vi "校准设置页.vi"() -> ()   [LabVIEW 2016, in "斯坦道CODMn.lvlib"]
uses:
  <vilib>/Analysis/6fits.llb/Curve Fitting Criteria.ctl
  <vilib>/Analysis/NI_AALPro.lvlib
  <vilib>/ptbypt/NI_PtbyPt.lvlib
panel:
  in  "读取公式":bool
  in  "历史数据导入":T1(radio)
  out "校准任务":bool
  in  "二次方程2":cluster{"K":dbl, "B":dbl, "x^2":dbl} {"x^2" format="%#.6g"; "K" format="%#.6g"; "B" format="%#.6g"}
  in  "公式切换阈值滴定数(0~9999)":dbl
  out "校准状态":T2(ring)
  out "模型刷新":bool
  in  "校准按钮":T1(radio)
  in  "校准导入":bool
  in  "曲线模型":T3={"标液浓度1"=0.0, "测量吸光度1"=0.0, "样品1启用"=FALSE, "标液浓度2"=0.0, "测量吸光度2"=0.0, "样品2启用"=FALSE, "标液浓度3"=0.0, "测量吸光度3"=0.0, "样品3启用"=FALSE, "标液浓度4"=0.0, "测量吸光度4"=0.0, "样品4启用"=FALSE, "标液浓度5"=0.0, "测量吸光度5"=0.0, "样品5启用"=FALSE, "模型"=enum."线性", "精度"=4.0, "XY图"=[], "拟合公式"="", "r^2"=0.0, "标样一校准时间"=timestamp(0 s since 1904-01-01), "标样二校准时间"=timestamp(0 s since 1904-01-01), "标样三校准时间"=timestamp(0 s since 1904-01-01), "标样四校准时间"=timestamp(0 s since 1904-01-01), "标样五校准时间"=timestamp(0 s since 1904-01-01), "二次方程"={"K"=0.0, "B"=0.0, "x^2"=0.0}, "标定时间"=timestamp(0 s since 1904-01-01), "拟合公式 2"="", "r^2 2"=0.0} {"r^2 2" format="%.7f"; "标定时间" format="%<%Y/%m/%d %H:%M:%S>T"; "二次方程"."x^2" format="%#.6g"; "二次方程"."K" format="%#.6g"; "二次方程"."B" format="%#.6g"; "标样五校准时间" format="%<%Y/%m/%d %H:%M:%S>T"; "标样四校准时间" format="%<%Y/%m/%d %H:%M:%S>T"; "标样三校准时间" format="%<%Y/%m/%d %H:%M:%S>T"; "标样二校准时间" format="%<%Y/%m/%d %H:%M:%S>T"; "标样一校准时间" format="%<%Y/%m/%d %H:%M:%S>T"; "r^2" format="%.7f"; "测量吸光度5" format="%#.6f"; "测量吸光度4" format="%#.6f"; "测量吸光度3" format="%#.6f"; "测量吸光度2" format="%#.6f"; "测量吸光度1" format="%#.6f"}
  in  "测量模式":T4(ring)
  in  "参数下拉列表":u16(ring) items=["CODMn"=21]
  in  "量程下拉列表":enum16{"低量程", "高量程"}(ring)
  # "校准时间"
  # "标液浓度"
  # "滴定数"
  # "标液一"
  # "标液二"
  # "标液三"
  # "零点"
  # "跨度"
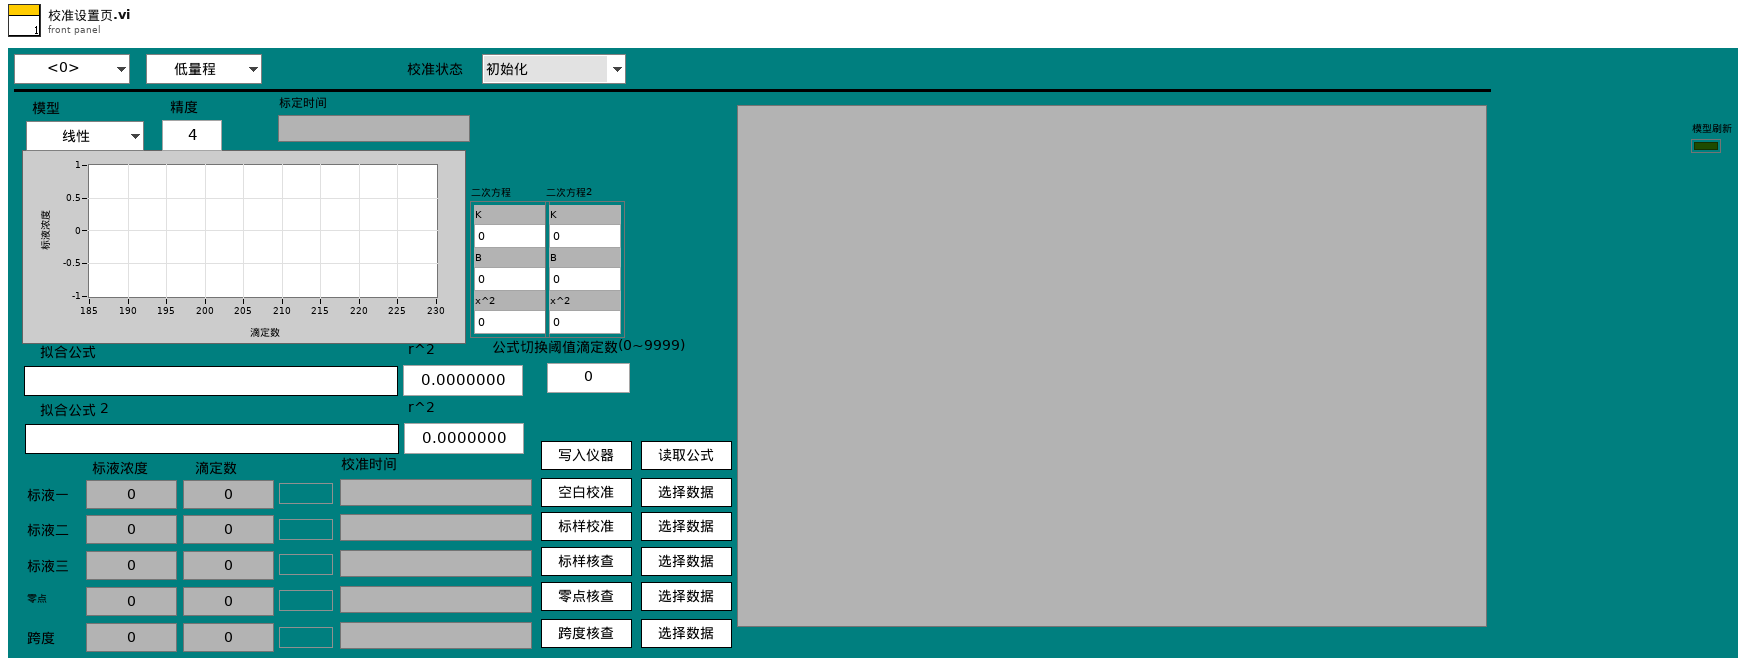
[diagram p1: front panel]
types:
  T1 = enum32{"未选择", "空白校准", "标样校准", "标样核查", "零点核查", "跨度核查"}
  T2 = enum16{"初始化", "解析数据", "判断任务类型", "执行测试任务", "等待测试任务完成", "获取测试数据", "任务结束判定", "计算公式", "结束"}
  T3 = cluster{"标液浓度1":dbl, "测量吸光度1":dbl, "样品1启用":bool, "标液浓度2":dbl, "测量吸光度2":dbl, "样品2启用":bool, "标液浓度3":dbl, "测量吸光度3":dbl, "样品3启用":bool, "标液浓度4":dbl, "测量吸光度4":dbl, "样品4启用":bool, "标液浓度5":dbl, "测量吸光度5":dbl, "样品5启用":bool, "模型":enum32{"线性", "多项式", "折线"}, "精度":dbl, "XY图":cluster{"X Values":dbl[], "Y Values":dbl[]}[], "拟合公式":string, "r^2":dbl, "标样一校准时间":timestamp, "标样二校准时间":timestamp, "标样三校准时间":timestamp, "标样四校准时间":timestamp, "标样五校准时间":timestamp, "二次方程":cluster{"K":dbl, "B":dbl, "x^2":dbl}, "标定时间":timestamp, "拟合公式 2":string, "r^2 2":dbl}
  T4 = enum16{"", "水样测量", "标样核查", "零点核查", "跨度核查", "空白测试", "平行样测试", "加标回收", "空白校准", "标样校准"}
  T5 = typedef "斯坦道CODMn.lvlib/校准任务.ctl" = cluster{"id":u16, "任务类型":enum16{"未选择", "空白校准", "标样校准", "标样核查", "零点核查", "跨度核查"}, "量程下拉列表":enum16{"低量程", "高量程"}, "状态":enum16{"已执行", "待执行", "执行中", "停止"}, "标液浓度":dbl, "吸光值":dbl, "校准时间":timestamp, "报警状态":enum16{"正常数据", "报警数据"}}
  T6 = cluster{"数组 2[0]":sgl, "数组 2[1]":sgl, "数组 2[2]":sgl, "数组 2[3]":sgl, "数组 2[4]":sgl, "数组 2[5]":sgl, "数组 2[6]":sgl, "数组 2[7]":sgl, "数组 2[8]":sgl, "数组 2[9]":sgl, "数组 2[10]":sgl, "数组 2[11]":sgl, "数组 2[12]":sgl, "数组 2[13]":sgl, "数组 2[14]":sgl, "数组 2[15]":sgl, "数组 2[16]":sgl, "数组 2[17]":sgl, "数组 2[18]":sgl, "数组 2[19]":sgl, "数组 2[20]":sgl, "数组 2[21]":sgl, "数组 2[22]":sgl, "数组 2[23]":sgl, "数组 2[24]":sgl, "数组 2[25]":sgl, "数组 2[26]":sgl, "数组 2[27]":sgl, "数组 2[28]":sgl, "数组 2[29]":sgl, "数组 2[30]":sgl, "数组 2[31]":sgl, "数组 2[32]":sgl, "数组 2[33]":sgl, "数组 2[34]":sgl, "数组 2[35]":sgl, "数组 2[36]":sgl, "数组 2[37]":sgl, "数组 2[38]":sgl, "数组 2[39]":sgl, "数组 2[40]":sgl, "数组 2[41]":sgl}
  T7 = cluster{"标液浓度1":dbl, "测量吸光度1":dbl, "样品1启用":bool, "标液浓度2":dbl, "测量吸光度2":dbl, "样品2启用":bool, "标液浓度3":dbl, "测量吸光度3":dbl, "样品3启用":bool, "标液浓度4":dbl, "测量吸光度4":dbl, "样品4启用":bool, "标液浓度5":dbl, "测量吸光度5":dbl, "样品5启用":bool, "模型":enum32{"线性", "多项式", "折线"}, "精度":dbl, "XY图":cluster{"X Values":dbl[], "Y Values":dbl[]}[], "拟合公式":string, "r^2":dbl, "标样一校准时间":timestamp, "标样二校准时间":timestamp, "标样三校准时间":timestamp, "标样四校准时间":timestamp, "标样五校准时间":timestamp, "二次方程":cluster{"c":dbl, "x":dbl, "x^2":dbl}, "标定时间":timestamp, "拟合公式 2":string, "r^2 2":dbl}[][]
  T8 = cluster{"标液浓度1":dbl, "测量吸光度1":dbl, "样品1启用":bool, "标液浓度2":dbl, "测量吸光度2":dbl, "样品2启用":bool, "标液浓度3":dbl, "测量吸光度3":dbl, "样品3启用":bool, "标液浓度4":dbl, "测量吸光度4":dbl, "样品4启用":bool, "标液浓度5":dbl, "测量吸光度5":dbl, "样品5启用":bool, "模型":enum32{"线性", "多项式", "折线"}, "精度":dbl, "XY图":cluster{"X Values":dbl[], "Y Values":dbl[]}[], "拟合公式":string, "r^2":dbl, "标样一校准时间":timestamp, "标样二校准时间":timestamp, "标样三校准时间":timestamp, "标样四校准时间":timestamp, "标样五校准时间":timestamp, "二次方程":cluster{"c":dbl, "x":dbl, "x^2":dbl}, "标定时间":timestamp, "拟合公式 2":string, "r^2 2":dbl}
  T9 = typedef "NI_AALPro.lvlib/Curve Fitting Criteria.ctl" = u16
  T10 = enum32{"Bad", "Idle", "Run top level", "Running"}
  T11 = cluster{"时间":timestamp, "标液值":dbl, "检测值":dbl, "吸光值":dbl}
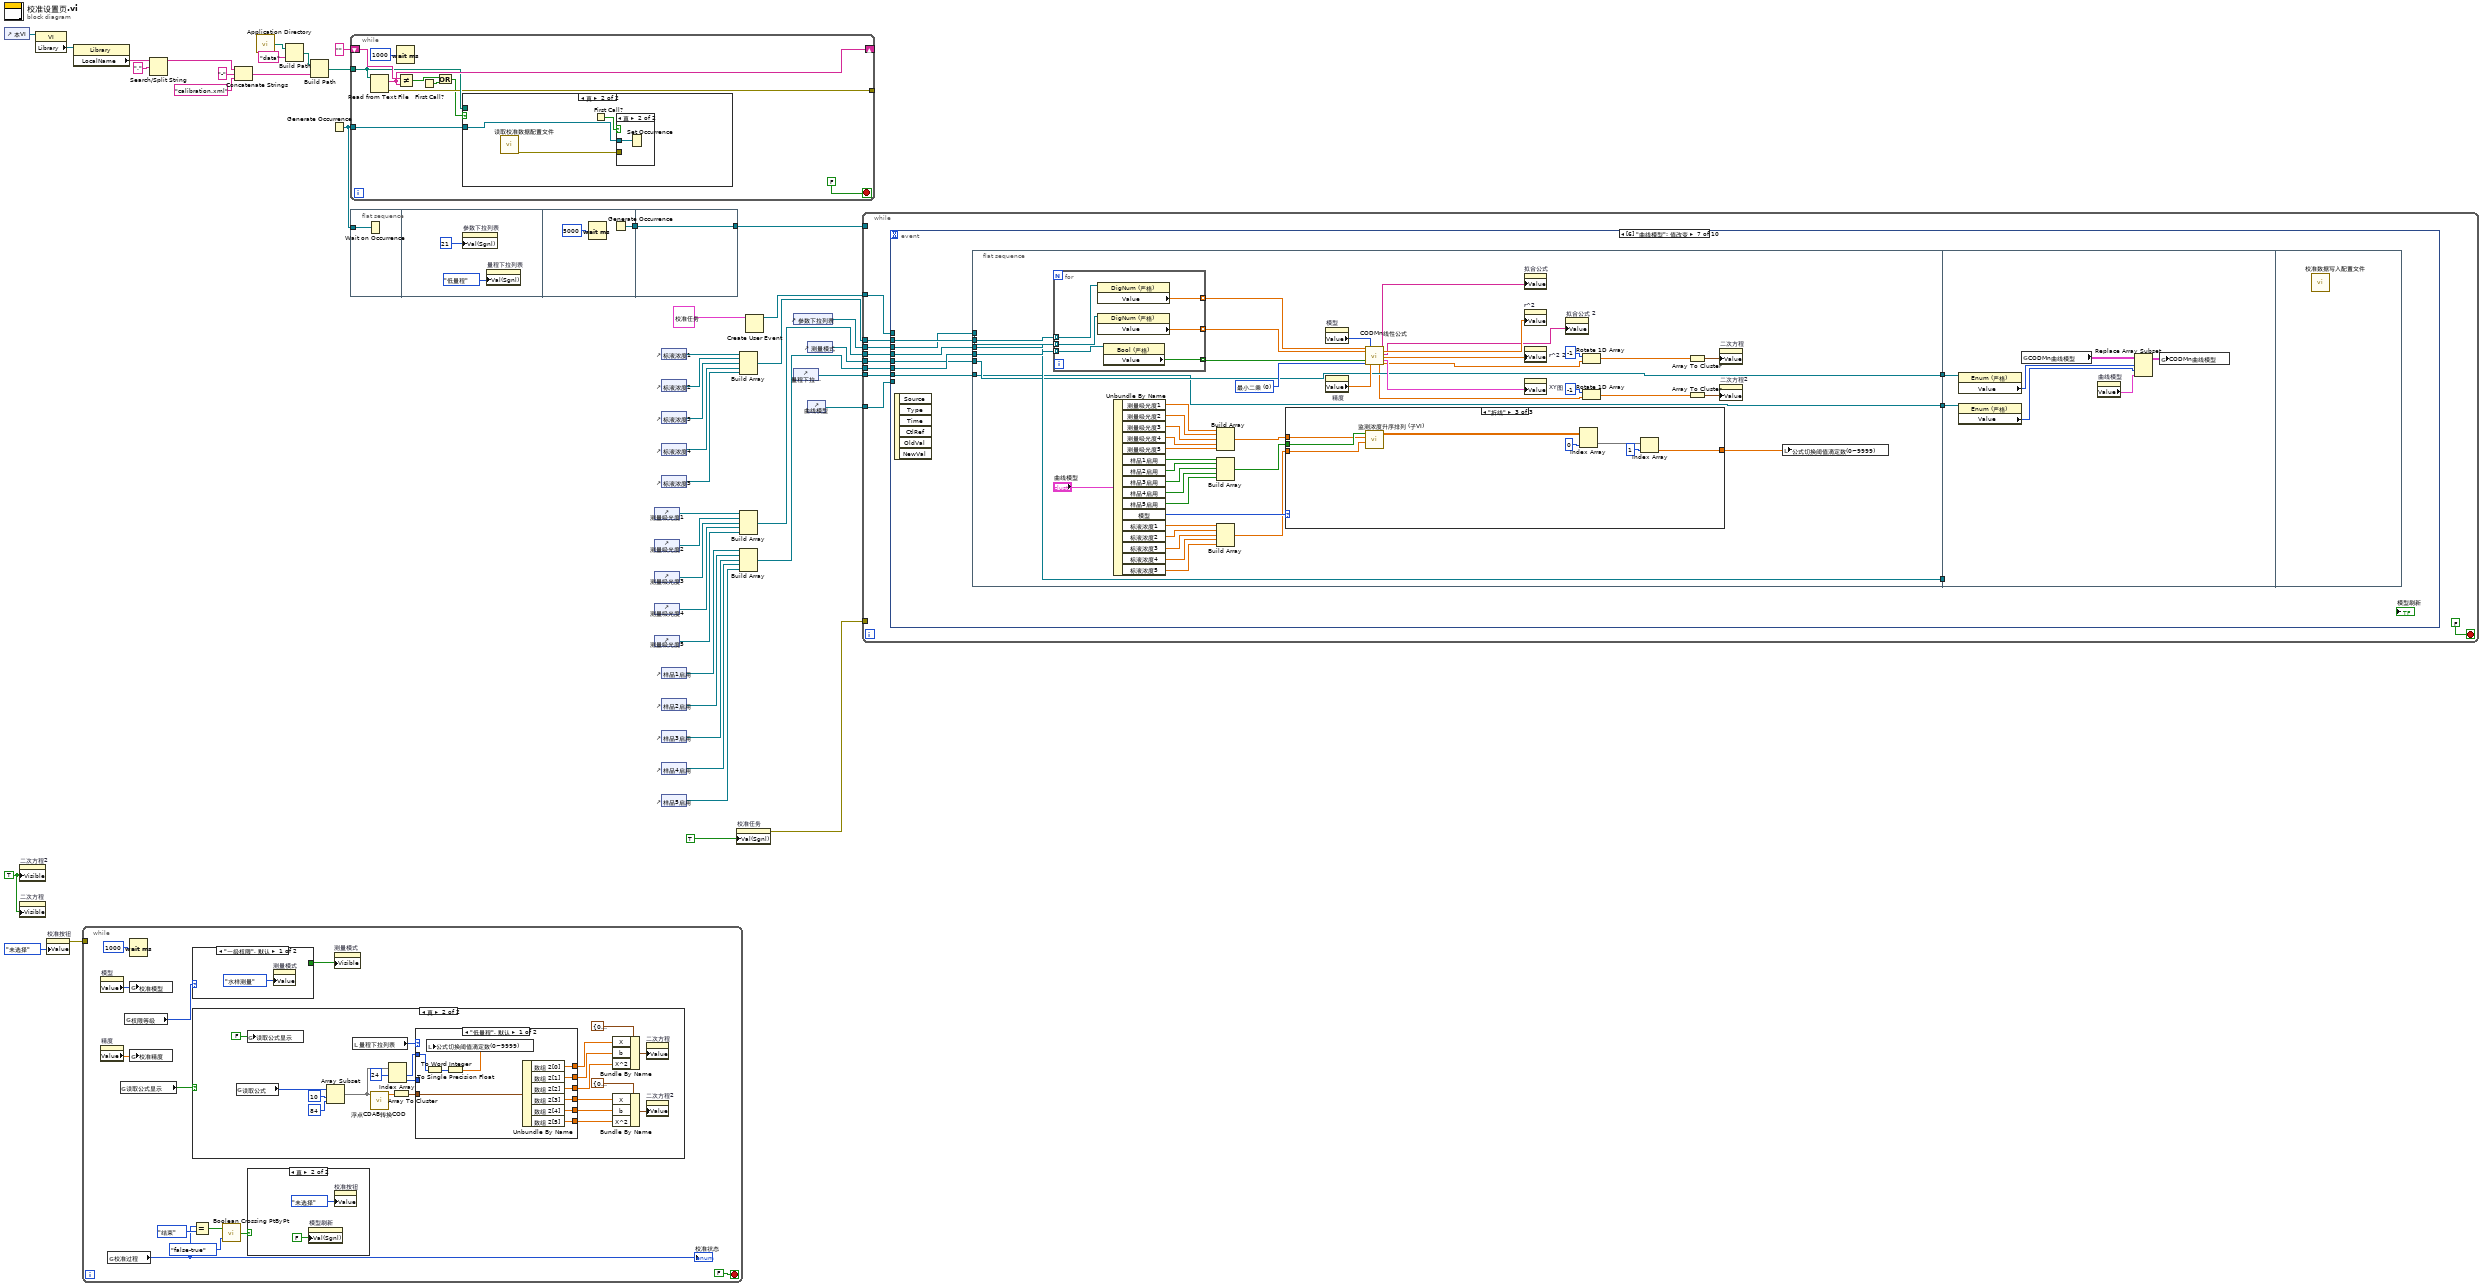
[diagram p0: block diagram]
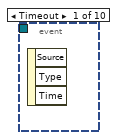
[diagram p4: hidden frame]
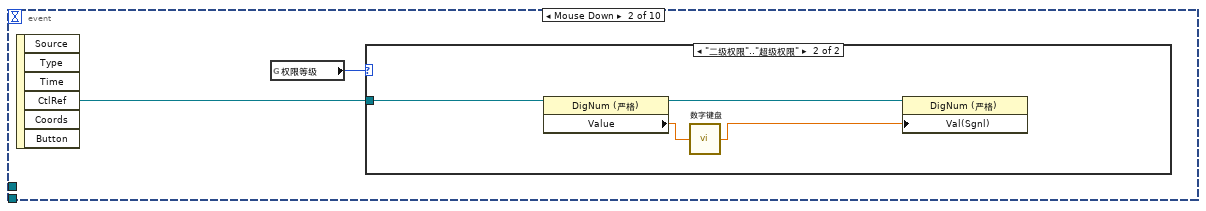
[diagram p5: hidden frame]
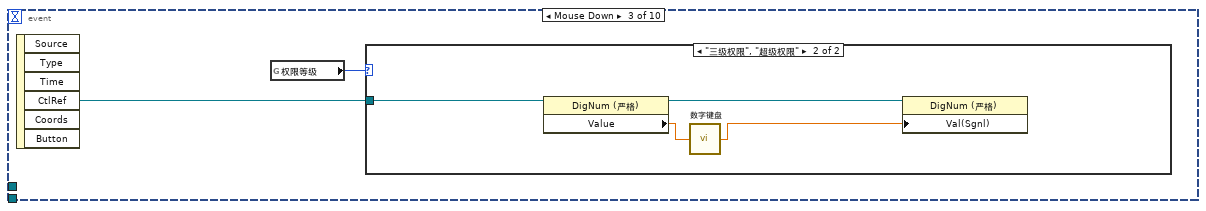
[diagram p7: hidden frame]
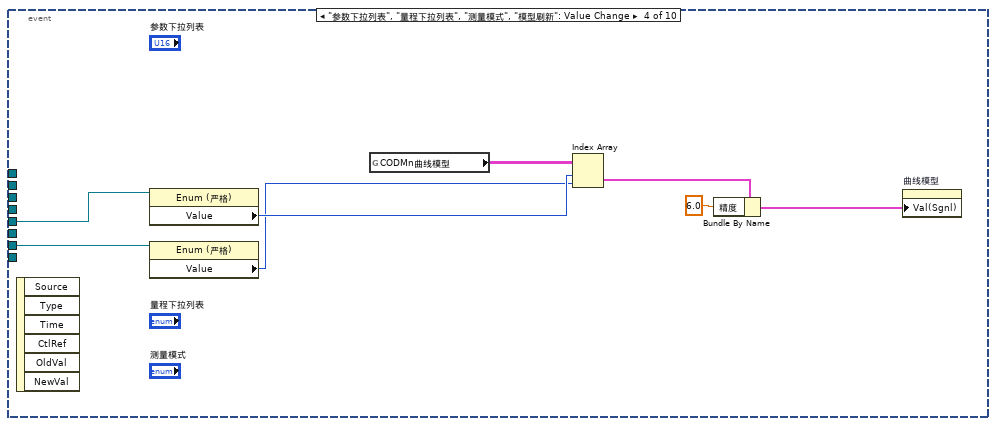
[diagram p9: hidden frame]
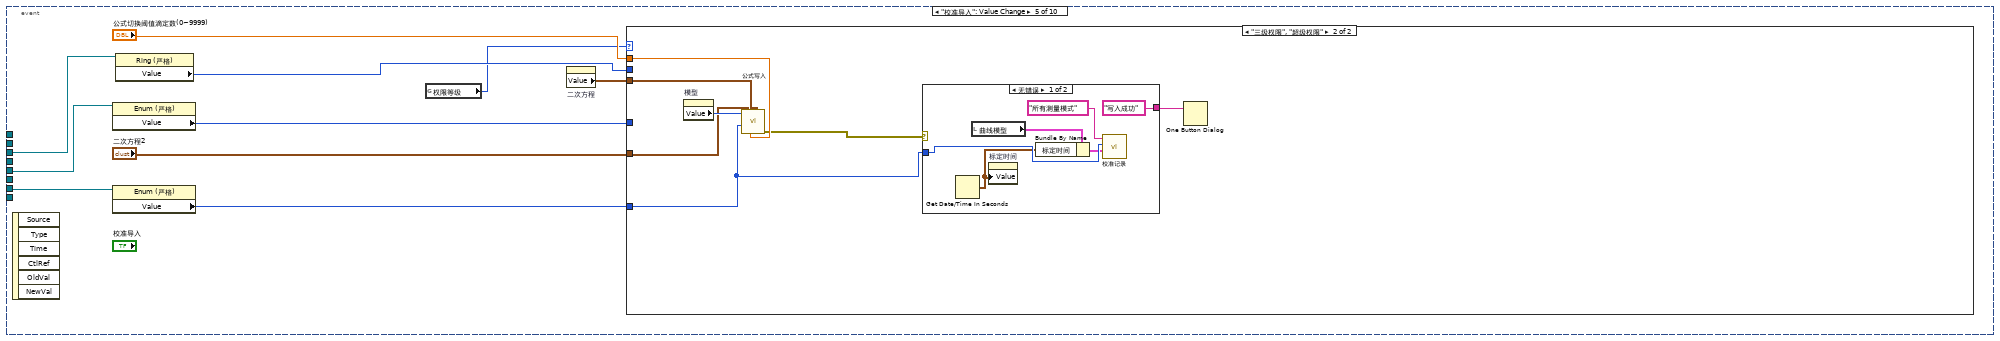
[diagram p10: hidden frame]
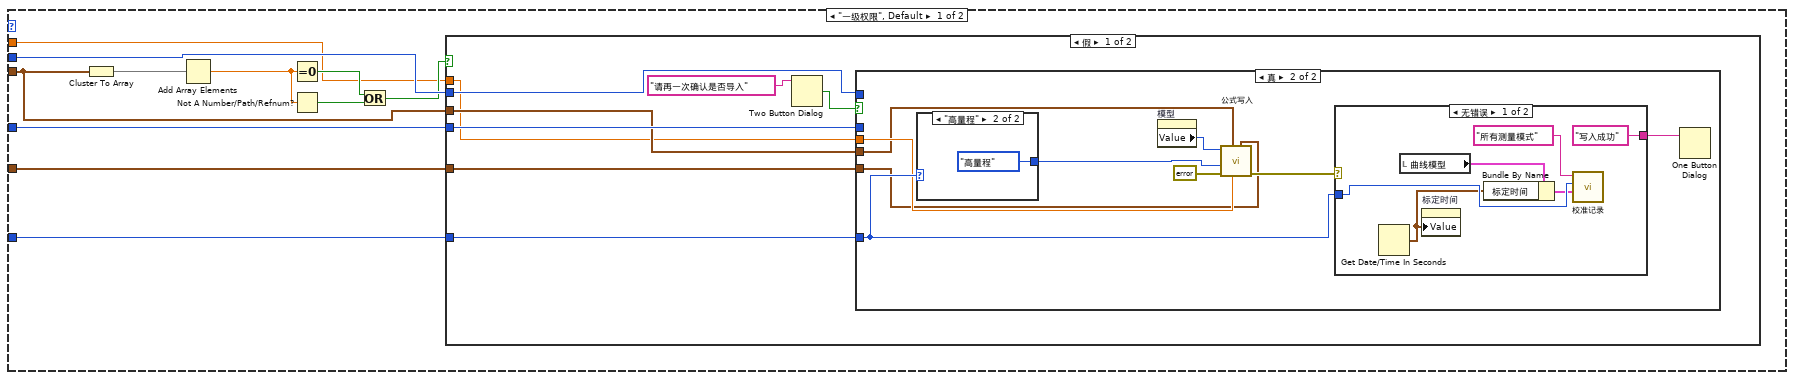
[diagram p11: hidden frame]
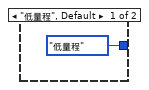
[diagram p13: hidden frame]
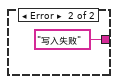
[diagram p14: hidden frame]
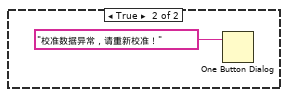
[diagram p15: hidden frame]
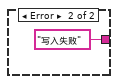
[diagram p16: hidden frame]
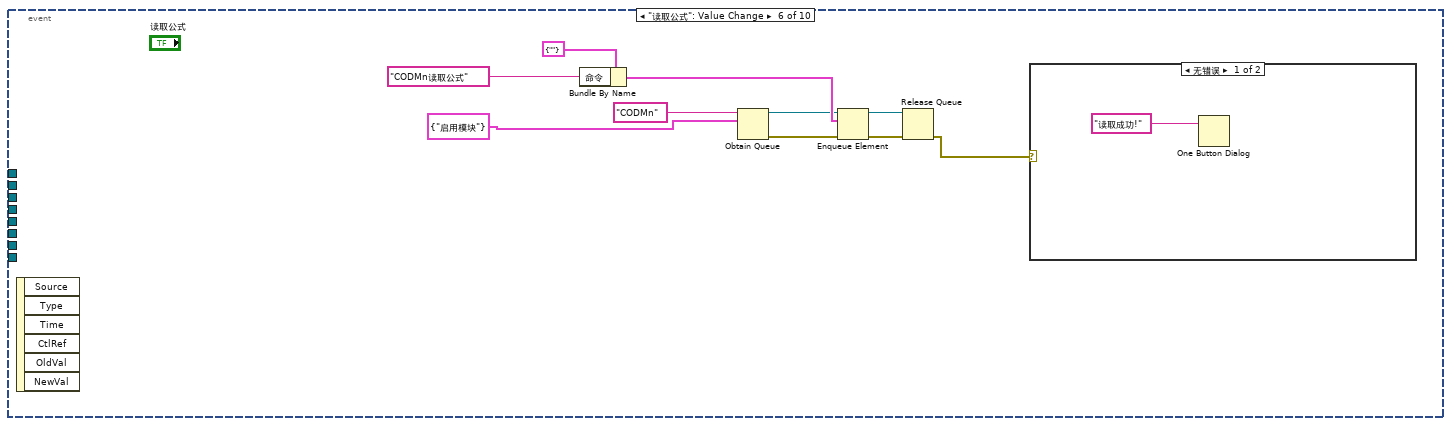
[diagram p17: hidden frame]
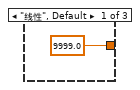
[diagram p19: hidden frame]
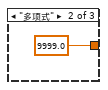
[diagram p20: hidden frame]
diagram:
  w2 = TRUE ("可见")
  n1 = control-ref of="本VI"() -> (w9:refnum<vi>)
  n2 = property on="二次方程2" class="Clust (严格)"("Visible"=w2) -> ()  [unwired: 2 in, 2 out]
  n3 = property on="二次方程" class="Clust (严格)"("Visible"=w2) -> ()  [unwired: 2 in, 2 out]
  n4 = property class="VI"(reference=w9) -> ("Library"=w18:refnum<vi>)  [unwired: 1 in, 2 out]
  n5 = property on="校准按钮" class="RadioBtnsControl (严格)"("Value"=T1."未选择" ("校准按钮")) -> (error out=w1:errorcluster)  [unwired: 2 in, 1 out]
  n6 = property class="Library"(reference=w18) -> ("LocalName"=w16:string)  [unwired: 1 in, 2 out]
  n7 = while {
    tunnel: w1 -> [_]
    stop <- FALSE stop-if-true
    n8 = property on="模型" class="Enum (严格)"() -> ("Value"=w49:enum32{"线性", "多项式", "折线"})  [unwired: 2 in, 2 out]
    n9 = property on="精度" class="DigNum (严格)"() -> ("Value"=w48:dbl)  [unwired: 2 in, 2 out]
    n10 = global read "校准数据全局变量.vi" "校准过程"() -> (w50:T2)
    "校准状态" <- w50
    n11 = global read "COD内部交互全局.vi" "读取公式显示"() -> (w46:bool)
    n12 = global read "CODMN外部API.vi" "权限等级"() -> (w47:enum16{"一级权限", "二级权限", "三级权限", "超级权限"})
    n13 = Wait (ms)(milliseconds to wait=u32 1000 ("等待时间（毫秒）")) -> ()  [unwired: 1 out]
    n14 = global write "校准数据全局变量.vi" "校准模型"(w49) -> ()
    n15 = global write "校准数据全局变量.vi" "校准精度"(w48) -> ()
    n16 = case shown="\"一级权限\", 默认" w47 {
      tunnel: [_ TRUE ("可见")] -> w55
      frame "一级权限", Default {
        n17 = property on="测量模式" class="Enum (严格)"("Value"=T4."水样测量" ("测量模式")) -> ()  [unwired: 2 in, 2 out]
      }
      frame "三级权限", "超级权限" {
      }
    }
    n18 = case shown="真" w46 {
      frame False {
      }
      frame True {
        n19 = global read "COD内部交互全局.vi" "读取公式"() -> (w72:u16[])
        n20 = global write "COD内部交互全局.vi" "读取公式显示"(FALSE ("读取公式显示")) -> ()
        n21 = Array Subset(array=w72, index=10 ("索引"), length=84 ("长度")) -> (w74:u16[])
        n22 = local read "量程下拉列表"() -> (w71:enum16{"低量程", "高量程"})
        n23 = call "浮点CDAB转换COD.vi"("数组"=w74) -> ("数组 2"=w77:sgl[])  [unwired: 10 in]
        n24 = Index Array(array=w74, index #1=24 ("索引")) -> (element #1=w68:u16, element #2=w69:u16)  [unwired: 1 in]
        n25 = Array To Cluster(array=w77) -> (cluster=w70:T6)
        n26 = case shown="\"低量程\", 默认" w71 {
          tunnel: w70 -> [w88 w98]
          tunnel: w69 -> [_ _]
          tunnel: w68 -> [w80 w90]
          tunnel: [w87 w97] -> w65
          tunnel: [w86 w96] -> w64
          tunnel: [w85 w95] -> w63
          tunnel: [w84 w94] -> w62
          tunnel: [w83 w93] -> w61
          tunnel: [w82 w92] -> w60
          frame "低量程", Default {
            n27 = To Word Integer(number=w80) -> (16bit integer=w81:i16)
            n28 = To Single Precision Float(number=w81) -> (single precision float=w79:sgl)
            n29 = local write "公式切换阈值滴定数(0~9999)"(w79) -> ()
            n30 = Unbundle By Name(w88) -> ("数组 2[0]"=w87:sgl, "数组 2[1]"=w86:sgl, "数组 2[2]"=w85:sgl, "数组 2[3]"=w84:sgl, "数组 2[4]"=w83:sgl, "数组 2[5]"=w82:sgl)
          }
          frame "高量程" {
            n31 = To Word Integer(number=w90) -> (16bit integer=w91:i16)
            n32 = To Single Precision Float(number=w91) -> (single precision float=w89:sgl)
            n33 = local write "公式切换阈值滴定数(0~9999)"(w89) -> ()
            n34 = Unbundle By Name(w98) -> ("数组 2[6]"=w97:sgl, "数组 2[7]"=w96:sgl, "数组 2[8]"=w95:sgl, "数组 2[9]"=w94:sgl, "数组 2[10]"=w93:sgl, "数组 2[11]"=w92:sgl)
          }
        }
        n35 = Bundle By Name(cluster=cluster{"X":dbl, "b":dbl, "X^2":dbl} {"X"=0.0, "b"=0.0, "X^2"=0.0} ("方程系数"), "X"=w65, "b"=w64, "X^2"=w63) -> (w59:cluster{"X":dbl, "b":dbl, "X^2":dbl})
        n36 = Bundle By Name(cluster=cluster{"X":dbl, "b":dbl, "X^2":dbl} {"X"=0.0, "b"=0.0, "X^2"=0.0} ("方程系数"), "X"=w62, "b"=w61, "X^2"=w60) -> (w58:cluster{"X":dbl, "b":dbl, "X^2":dbl})
        n37 = property on="二次方程" class="Clust (严格)"("Value"=w59) -> ()  [unwired: 2 in, 2 out]
        n38 = property on="二次方程2" class="Clust (严格)"("Value"=w58) -> ()  [unwired: 2 in, 2 out]
      }
    }
    n39 = Equal?(x=w50, y=T2."结束" ("校准过程")) -> (x = y?=w54:bool)
    n40 = call <vilib>:"Boolean Crossing PtByPt.vi"("direction"=enum16{"either", "false-true", "true-false"}."false-true", "input"=w54) -> ("crossing"=w52:bool)  [unwired: 1 in]
    n41 = case shown="真" w52 {
      frame False {
      }
      frame True {
        n42 = property on="模型刷新" class="Bool (严格)"("Val(Sgnl)"=FALSE ("值(信号)")) -> ()  [unwired: 2 in, 2 out]
        n43 = property on="校准按钮" class="RadioBtnsControl (严格)"("Value"=T1."未选择" ("校准按钮")) -> ()  [unwired: 2 in, 2 out]
      }
    }
    n44 = property on="测量模式" class="Enum (严格)"("Visible"=w55) -> ()  [unwired: 2 in, 2 out]
  }
  n45 = Search/Split String(string=w16, search string/char (-)="." ("搜索字符串/字符(-)")) -> (substring before match=w14:string)  [unwired: 1 in, 2 out]
  n46 = Concatenate Strings(w14, "-" ("字符串"), "calibration.xml" ("名称或相对路径")) -> (w11:string)
  n47 = call <vilib>:"Application Directory.vi"() -> ("Application Directory"=w19:path)
  n48 = Build Path(base path=w19, name or relative path="data" ("名称或相对路径")) -> (appended path=w17:path)
  n49 = Build Path(base path=w17, name or relative path=w11) -> (appended path=w10:path)
  n50 = Generate Occurrence() -> (w7:refnum<k4>)
  n51 = while {
    shift-right: [w110] -> _
    shift-left: "" -> [w111]
    tunnel: w10 -> [w109]
    tunnel: [w107] -> _
    tunnel: w7 -> [w103]
    stop <- FALSE stop-if-true
    n52 = Read from Text File(file (use dialog)=w109) -> (text=w110:string, error out=w107:errorcluster)  [unwired: 3 in, 2 out]
    n53 = Wait (ms)(milliseconds to wait=u32 1000 ("等待时间（毫秒）")) -> ()  [unwired: 1 out]
    n54 = Not Equal?(x=w111, y=w110) -> (x != y?=w105:bool)
    n55 = First Call?() -> (First Call?: T/F=w106:bool)
    n56 = Or(x=w105, y=w106) -> (x .or. y?=w104:bool)
    n57 = case shown="真" w104 {
      tunnel: w109 -> [_ _]
      tunnel: w103 -> [_ w114]
      frame False {
      }
      frame True {
        n58 = call "读取校准数据配置文件.vi"() -> ("错误输出"=w113:errorcluster)  [unwired: 11 in]
        n59 = First Call?() -> (First Call?: T/F=w115:bool)
        n60 = case shown="真" w115 {
          tunnel: w114 -> [_ w116]
          tunnel: w113 -> [_ _]
          frame False {
          }
          frame True {
            n61 = Set Occurrence(w116) -> ()
          }
        }
      }
    }
  }
  n62 = flat-sequence {
    tunnel: w7 -> [w117]
    tunnel: [w121] -> w45
    tunnel: [w122] -> w44
    tunnel: w45 -> [w122]
    frame #0 {
      n63 = Wait on Occurrence(2:w117) -> ()  [unwired: 2 in, 1 out]
    }
    frame #1 {
      n64 = property on="参数下拉列表" class="Ring (严格)"("Val(Sgnl)"=u16 21 ("值(信号)")) -> ()  [unwired: 2 in, 2 out]
      n65 = property on="量程下拉列表" class="Enum (严格)"("Val(Sgnl)"=enum16{"低量程", "高量程"}."低量程" ("值(信号)")) -> ()  [unwired: 2 in, 2 out]
    }
    frame #2 {
      n66 = Wait (ms)(milliseconds to wait=u32 5000 ("等待时间（毫秒）")) -> ()  [unwired: 1 out]
      n67 = Generate Occurrence() -> (w121:refnum<k4>)
    }
    frame #3 {
    }
  }
  n68 = control-ref of="测量吸光度1"() -> (w32:refnum<vi>)
  n69 = control-ref of="测量吸光度2"() -> (w33:refnum<vi>)
  n70 = control-ref of="测量吸光度3"() -> (w34:refnum<vi>)
  n71 = control-ref of="测量吸光度4"() -> (w35:refnum<vi>)
  n72 = control-ref of="测量吸光度5"() -> (w36:refnum<vi>)
  n73 = control-ref of="标液浓度1"() -> (w30:refnum<vi>)
  n74 = control-ref of="标液浓度2"() -> (w29:refnum<vi>)
  n75 = control-ref of="标液浓度3"() -> (w28:refnum<vi>)
  n76 = control-ref of="标液浓度4"() -> (w27:refnum<vi>)
  n77 = control-ref of="标液浓度5"() -> (w26:refnum<vi>)
  n78 = control-ref of="样品1启用"() -> (w42:refnum<vi>)
  n79 = control-ref of="样品2启用"() -> (w41:refnum<vi>)
  n80 = control-ref of="样品3启用"() -> (w40:refnum<vi>)
  n81 = control-ref of="样品4启用"() -> (w39:refnum<vi>)
  n82 = control-ref of="样品5启用"() -> (w38:refnum<vi>)
  n83 = property on="校准任务" class="Bool (严格)"("Val(Sgnl)"=TRUE ("值(信号)")) -> (error out=w5:errorcluster)  [unwired: 2 in, 1 out]
  n84 = Build Array(w30, w29, w28, w27, w26) -> (w25:refnum<vi>[])
  n85 = Build Array(w32, w33, w34, w35, w36) -> (w31:refnum<vi>[])
  n86 = Build Array(w42, w41, w40, w39, w38) -> (w37:refnum<vi>[])
  n87 = Create User Event(user event datatype=T5 {"id"=0, "任务类型"=enum."未选择", "量程下拉列表"=enum."低量程", "状态"=enum."已执行", "标液浓度"=0.0, "吸光值"=0.0, "校准时间"=timestamp(0 s since 1904-01-01), "报警状态"=enum."正常数据"} ("校准任务")) -> (user event=w3:refnum<user-event>)  [unwired: 1 in, 1 out]
  n88 = control-ref of="参数下拉列表"() -> (w43:refnum<vi>)
  n89 = control-ref of="量程下拉列表"() -> (w23:refnum<vi>)
  n90 = control-ref of="测量模式"() -> (w24:refnum<vi>)
  n91 = control-ref of="曲线模型"() -> (w21:refnum<vi>)
  n92 = while {
    tunnel: w44 -> [_]
    tunnel: w43 -> [w130]
    tunnel: w37 -> [w129]
    tunnel: w31 -> [w128]
    tunnel: w25 -> [w127]
    tunnel: w24 -> [w126]
    tunnel: w23 -> [w125]
    tunnel: w21 -> [w124]
    tunnel: w5 -> [_]
    tunnel: w3 -> [w123]
    stop <- FALSE stop-if-true
    n93 = event shown="[6] \"曲线模型\": 值改变" {
      selector: _ -> [_ _ _ _ _ _ _ _ _ _]
      dyn-events: _ -> [_ _ _ _ _ _ _ _ _ _]
      timeout: _ -> [_ _ _ _ _ _ _ _ _ _]
      tunnel: w130 -> [_ _ _ _ w161 _ w229 _ w331 w358]
      tunnel: w129 -> [_ _ _ _ _ _ w233 _ _ _]
      tunnel: w128 -> [_ _ _ _ _ _ w232 _ _ _]
      tunnel: w127 -> [_ _ _ _ _ _ w231 _ _ _]
      tunnel: w126 -> [_ _ _ w151 w159 _ w227 _ w326 w353]
      tunnel: w125 -> [_ _ _ w150 w157 _ w225 _ w330 w357]
      tunnel: w124 -> [_ _ _ _ _ _ _ _ w324 _]
      tunnel: w123 -> [_ _ _ _ _ _ _ w304 w323 w352]
      event Timeout {
        n94 = event-data() -> ()  [unwired: 1 in, 3 out]
      }
      event "曲线模型.标液浓度1", "曲线模型.标液浓度2", "曲线模型.标液浓度3", "曲线模型.标液浓度4", "曲线模型.标液浓度5", "曲线模型.精度": Mouse Down {
        n95 = event-data() -> ("CtlRef"=w133:refnum<vi>)  [unwired: 1 in, 5 out]
        n96 = global read "CODMN外部API.vi" "权限等级"() -> (w132:enum16{"一级权限", "二级权限", "三级权限", "超级权限"})
        n97 = case shown="\"二级权限\"..\"超级权限\"" w132 {
          tunnel: w133 -> [_ w137]
          frame "一级权限", Default {
          }
          frame "二级权限".."超级权限" {
            n98 = property class="DigNum (严格)"(reference=w137) -> (reference out=w135:refnum<vi>, "Value"=w136:dbl)  [unwired: 1 in, 1 out]
            n99 = call "数字键盘.vi"("OldNumber"=w136) -> ("NewNumber"=w134:sgl)
            n100 = property class="DigNum (严格)"(reference=w135, "Val(Sgnl)"=w134) -> ()  [unwired: 1 in, 2 out]
          }
        }
      }
      event "曲线模型.测量吸光度1", "曲线模型.测量吸光度2", "曲线模型.测量吸光度3", "曲线模型.测量吸光度4", "曲线模型.测量吸光度5": Mouse Down {
        n101 = event-data() -> ("CtlRef"=w139:refnum<vi>)  [unwired: 1 in, 5 out]
        n102 = global read "CODMN外部API.vi" "权限等级"() -> (w138:enum16{"一级权限", "二级权限", "三级权限", "超级权限"})
        n103 = case shown="\"三级权限\", \"超级权限\"" w138 {
          tunnel: w139 -> [_ w143]
          frame "一级权限", Default {
          }
          frame "三级权限", "超级权限" {
            n104 = property class="DigNum (严格)"(reference=w143) -> (reference out=w141:refnum<vi>, "Value"=w142:dbl)  [unwired: 1 in, 1 out]
            n105 = call "数字键盘.vi"("OldNumber"=w142) -> ("NewNumber"=w140:sgl)
            n106 = property class="DigNum (严格)"(reference=w141, "Val(Sgnl)"=w140) -> ()  [unwired: 1 in, 2 out]
          }
        }
      }
      event "参数下拉列表", "量程下拉列表", "测量模式", "模型刷新": Value Change {
        n107 = event-data() -> ()  [unwired: 1 in, 6 out]
        n108 = property class="Enum (严格)"(reference=w151) -> ("Value"=w148:T4)  [unwired: 1 in, 2 out]
        n109 = property class="Enum (严格)"(reference=w150) -> ("Value"=w147:enum16{"低量程", "高量程"})  [unwired: 1 in, 2 out]
        n110 = global read "校准数据全局变量.vi" "CODMn曲线模型"() -> (w149:T7)
        n111 = Index Array(array=w149, index (row)=w148, index (col)=w147) -> (element=w146:T8)
        n112 = Bundle By Name(cluster=w146, "精度"=6.0 ("值")) -> (w145:T8)
        n113 = property on="曲线模型" class="Clust (严格)"("Val(Sgnl)"=w145) -> ()  [unwired: 2 in, 2 out]
      }
      event "校准导入": Value Change {
        n114 = event-data() -> ()  [unwired: 1 in, 6 out]
        n115 = property class="Enum (严格)"(reference=w159) -> ("Value"=w158:T4)  [unwired: 1 in, 2 out]
        n116 = property class="Enum (严格)"(reference=w157) -> ("Value"=w156:enum16{"低量程", "高量程"})  [unwired: 1 in, 2 out]
        n117 = property class="Ring (严格)"(reference=w161) -> ("Value"=w160:u16)  [unwired: 1 in, 2 out]
        n118 = global read "CODMN外部API.vi" "权限等级"() -> (w153:enum16{"一级权限", "二级权限", "三级权限", "超级权限"})
        n119 = property on="二次方程" class="Clust (严格)"() -> ("Value"=w152:cluster{"K":dbl, "B":dbl, "x^2":dbl})  [unwired: 2 in, 2 out]
        n120 = case shown="\"三级权限\", \"超级权限\"" w153 {
          tunnel: w160 -> [w172 _]
          tunnel: w158 -> [w171 _]
          tunnel: w156 -> [w170 w200]
          tunnel: w152 -> [w164 w204]
          tunnel: "公式切换阈值滴定数(0~9999)" -> [w163 w205]
          tunnel: "二次方程2" -> [w162 w203]
          frame "一级权限", Default {
            n121 = Cluster To Array(cluster=w164) -> (array=w169:dbl[])
            n122 = Add Array Elements(numeric array=w169) -> (sum=w168:dbl)
            n123 = Equal To 0?(x=w168) -> (x = 0?=w166:bool)
            n124 = Not A Number/Path/Refnum?(number/path/refnum=w168) -> (NaN/Path/Refnum?=w167:bool)
            n125 = Or(x=w166, y=w167) -> (x .or. y?=w165:bool)
            n126 = case shown="假" w165 {
              tunnel: w172 -> [w180 _]
              tunnel: w171 -> [w179 _]
              tunnel: w170 -> [w178 _]
              tunnel: w164 -> [w175 _]
              tunnel: w163 -> [w174 _]
              tunnel: w162 -> [w173 _]
              frame False {
                n127 = Two Button Dialog(message="请再一次确认是否导入" ("消息")) -> (T button?=w176:bool)  [unwired: 2 in]
                n128 = case shown="真" w176 {
                  tunnel: w180 -> [_ _]
                  tunnel: w179 -> [_ _]
                  tunnel: w178 -> [_ w188]
                  tunnel: w175 -> [_ w181]
                  tunnel: w174 -> [_ w184]
                  tunnel: w173 -> [_ w182]
                  frame False {
                  }
                  frame True {
                    n129 = case shown="\"高量程\"" w188 {
                      tunnel: [enum16{"低量程", "高量程"}."低量程" ("量程选择") enum16{"低量程", "高量程"}."高量程" ("量程选择")] -> w185
                      frame "低量程", Default {
                      }
                      frame "高量程" {
                      }
                    }
                    n130 = property on="模型" class="Enum (严格)"() -> ("Value"=w183:enum32{"线性", "多项式", "折线"})  [unwired: 2 in, 2 out]
                    n131 = call "公式写入.vi"("公式 2"=w182, "公式切换阈值滴定数(0-9999)"=w184, "公式"=w181, "Error in"=errorcluster {"status"=FALSE, "code"=0, "source"=""} ("error out"), "量程选择"=w185, "模型"=w183) -> ("error out"=w187:errorcluster)  [unwired: 5 in]
                    n132 = case shown="无错误" w187 {
                      tunnel: ["写入成功" "写入失败"] -> w189
                      tunnel: w188 -> [w196 _]
                      frame No Error {
                        n133 = Get Date/Time In Seconds() -> (seconds since 1Jan1904=w193:timestamp)
                        n134 = local read "曲线模型"() -> (w194:T3)
                        n135 = property on="标定时间" class="AbsTime (严格)"("Value"=w193) -> ()  [unwired: 2 in, 2 out]
                        n136 = Bundle By Name(cluster=w194, "标定时间"=w193) -> (w192:T3)
                        n137 = call "校准记录.vi"("曲线模型"=w192, "量程"=w196, "测量模式"="所有测量模式") -> ()  [unwired: 8 in, 1 out]
                      }
                      frame Error {
                      }
                    }
                    n138 = One Button Dialog(message=w189) -> ()  [unwired: 1 in, 1 out]
                  }
                }
              }
              frame True {
                n139 = One Button Dialog(message="校准数据异常，请重新校准！" ("消息")) -> ()  [unwired: 1 in, 1 out]
              }
            }
          }
          frame "三级权限", "超级权限" {
            n140 = property on="模型" class="Enum (严格)"() -> ("Value"=w206:enum32{"线性", "多项式", "折线"})  [unwired: 2 in, 2 out]
            n141 = call "公式写入.vi"("公式 2"=w203, "公式切换阈值滴定数(0-9999)"=w205, "公式"=w204, "量程选择"=w200, "模型"=w206) -> ("error out"=w201:errorcluster)  [unwired: 6 in]
            n142 = case shown="无错误" w201 {
              tunnel: ["写入成功" "写入失败"] -> w202
              tunnel: w200 -> [w211 _]
              frame No Error {
                n143 = Get Date/Time In Seconds() -> (seconds since 1Jan1904=w208:timestamp)
                n144 = local read "曲线模型"() -> (w209:T3)
                n145 = property on="标定时间" class="AbsTime (严格)"("Value"=w208) -> ()  [unwired: 2 in, 2 out]
                n146 = Bundle By Name(cluster=w209, "标定时间"=w208) -> (w207:T3)
                n147 = call "校准记录.vi"("曲线模型"=w207, "量程"=w211, "测量模式"="所有测量模式") -> ()  [unwired: 8 in, 1 out]
              }
              frame Error {
              }
            }
            n148 = One Button Dialog(message=w202) -> ()  [unwired: 1 in, 1 out]
          }
        }
      }
      event "读取公式": Value Change {
        n149 = event-data() -> ()  [unwired: 1 in, 6 out]
        n150 = Bundle By Name(cluster=cluster{"命令":string} {"命令"=""} ("元素"), "命令"="CODMn读取公式" ("名称（未命名）")) -> (w221:cluster{"命令":string})
        n151 = Obtain Queue(name (unnamed)="CODMn" ("名称（未命名）"), element data type=cluster{"命令":string} {"命令"="启用模块"} ("元素")) -> (queue out=w217:refnum<queue>, error out=w218:errorcluster)  [unwired: 3 in, 1 out]
        n152 = Enqueue Element(queue=w217, element=w221, error in (no error)=w218) -> (queue out=w216:refnum<queue>, error out=w215:errorcluster)  [unwired: 1 in, 1 out]
        n153 = Release Queue(queue=w216, error in (no error)=w215) -> (error out=w214:errorcluster)  [unwired: 1 in, 2 out]
        n154 = case shown="无错误" w214 {
          frame No Error {
            n155 = One Button Dialog(message="读取成功!") -> ()  [unwired: 1 in, 1 out]
          }
          frame Error {
          }
        }
      }
      event "曲线模型": Value Change {
        n156 = event-data() -> ()  [unwired: 1 in, 6 out]
        n157 = flat-sequence {
          tunnel: w233 -> [w279]
          tunnel: w232 -> [w277]
          tunnel: w231 -> [w275]
          tunnel: [w267] -> w230
          tunnel: w229 -> [w267]
          tunnel: [w266] -> w228
          tunnel: w227 -> [w266]
          tunnel: [w265] -> w226
          tunnel: w225 -> [w265]
          tunnel: w230 -> [_]
          tunnel: w228 -> [w301]
          tunnel: w226 -> [w300]
          frame #0 {
            w271 = T9 0 items=["最小二乘", "最小绝对残差", "Bisquare"] ("method")
            n158 = for {
              tunnel: w279 -> [w295] mode=indexing
              tunnel: [w294] -> w278 mode=indexing
              tunnel: w277 -> [w293] mode=indexing
              tunnel: [w292] -> w276 mode=indexing
              tunnel: w275 -> [w291] mode=indexing
              tunnel: [w290] -> w274 mode=indexing
              n159 = property class="DigNum (严格)"(reference=w291) -> ("Value"=w290:dbl)  [unwired: 1 in, 2 out]
              n160 = property class="DigNum (严格)"(reference=w293) -> ("Value"=w292:dbl)  [unwired: 1 in, 2 out]
              n161 = property class="Bool (严格)"(reference=w295) -> ("Value"=w294:bool)  [unwired: 1 in, 2 out]
            }
            n162 = Unbundle By Name("曲线模型") -> ("测量吸光度1"=w263:dbl, "测量吸光度2"=w262:dbl, "测量吸光度3"=w261:dbl, "测量吸光度4"=w259:dbl, "测量吸光度5"=w260:dbl, "样品1启用"=w258:bool, "样品2启用"=w257:bool, "样品3启用"=w256:bool, "样品4启用"=w255:bool, "样品5启用"=w254:bool, "模型"=w248:enum32{"线性", "多项式", "折线"}, "标液浓度1"=w247:dbl, "标液浓度2"=w246:dbl, "标液浓度3"=w245:dbl, "标液浓度4"=w244:dbl, "标液浓度5"=w243:dbl)
            n163 = Build Array(w263, w262, w261, w259, w260) -> (w252:dbl[])
            n164 = Build Array(w258, w257, w256, w255, w254) -> (w253:bool[])
            n165 = Build Array(w247, w246, w245, w244, w243) -> (w242:dbl[])
            n166 = case shown="\"折线\"" w248 {
              tunnel: w253 -> [_ _ w287]
              tunnel: w252 -> [_ _ w286]
              tunnel: [9999.0 ("数值") 9999.0 ("数值") w288] -> w249
              tunnel: w242 -> [_ _ w285]
              frame "线性", Default {
              }
              frame "多项式" {
              }
              frame "折线" {
                n167 = call "监测浓度升序排列 (子VI).vi"("标液浓度"=w285, "滴定数"=w286, "启用"=w287) -> ("输出数组"=w284:dbl[][])  [unwired: 8 in]
                n168 = Index Array(array=w284, index (col)=0 ("禁用的索引 (列)")) -> (element=w282:dbl[])  [unwired: 1 in]
                n169 = Index Array(array=w282, index=1 ("索引")) -> (element=w288:dbl)
              }
            }
            n170 = property on="模型" class="Enum (严格)"() -> ("Value"=w273:enum32{"线性", "多项式", "折线"})  [unwired: 2 in, 2 out]
            n171 = property on="精度" class="DigNum (严格)"() -> ("Value"=w272:dbl)  [unwired: 2 in, 2 out]
            n172 = call "CODMn线性公式.vi"("标液浓度"=w274, "滴定数"=w276, "启用"=w278, "method"=w271, "模型"=w273, "精度"=w272) -> ("Polynomial Coefficients 2"=w239:dbl[], "拟合方程"=w270:string, "r^2"=w269:dbl, "拟合方程 2"=w251:string, "r^2 2"=w250:dbl, "XY图"=w268:cluster{"X Values":dbl[], "Y Values":dbl[]}[], "Polynomial Coefficients"=w235:dbl[])  [unwired: 7 in]
            n173 = property on="拟合公式" class="Str"("Value"=w270) -> ()  [unwired: 2 in, 2 out]
            n174 = property on="r^2" class="DigNum (严格)"("Value"=w269) -> ()  [unwired: 2 in, 2 out]
            n175 = property on="r^2 2" class="DigNum (严格)"("Value"=w250) -> ()  [unwired: 2 in, 2 out]
            n176 = property on="XY图" class="XYGraph (严格)"("Value"=w268) -> ()  [unwired: 2 in, 2 out]
            n177 = property on="拟合公式 2" class="Str"("Value"=w251) -> ()  [unwired: 2 in, 2 out]
            n178 = Rotate 1D Array(1:w235, 2:-1 ("n")) -> (0:w237:dbl[])
            n179 = Rotate 1D Array(1:w239, 2:-1 ("n")) -> (0:w241:dbl[])
            n180 = Array To Cluster(array=w237) -> (cluster=w234:cluster{"[0]":dbl, "[1]":dbl, "[2]":dbl})
            n181 = Array To Cluster(array=w241) -> (cluster=w238:cluster{"[0]":dbl, "[1]":dbl, "[2]":dbl})
            n182 = property on="二次方程" class="Clust (严格)"("Value"=w234) -> ()  [unwired: 2 in, 2 out]
            n183 = property on="二次方程2" class="Clust (严格)"("Value"=w238) -> ()  [unwired: 2 in, 2 out]
            n184 = local write "公式切换阈值滴定数(0~9999)"(w249) -> ()
          }
          frame #1 {
            n185 = property class="Enum (严格)"(reference=w301) -> ("Value"=w298:T4)  [unwired: 1 in, 2 out]
            n186 = property class="Enum (严格)"(reference=w300) -> ("Value"=w299:enum16{"低量程", "高量程"})  [unwired: 1 in, 2 out]
            n187 = global read "校准数据全局变量.vi" "CODMn曲线模型"() -> (w297:T7)
            n188 = property on="曲线模型" class="Clust (严格)"() -> ("Value"=w302:T3)  [unwired: 2 in, 2 out]
            n189 = Replace Array Subset(array=w297, new element=w302, index (row)=w298, index (col)=w299) -> (w296:T7)
            n190 = global write "校准数据全局变量.vi" "CODMn曲线模型"(w296) -> ()
          }
          frame #2 {
            n191 = call "校准数据写入配置文件.vi"() -> ()  [unwired: 11 in, 1 out]
          }
        }
      }
      event "校准任务": Value Change {
        n192 = event-data() -> ("NewVal"=w305:bool)  [unwired: 1 in, 5 out]
        n193 = invoke on="子面板" class="SubPnl" method="Remove VI"() -> (error out=w303:errorcluster)  [unwired: 3 in, 2 out]
        n194 = case shown="真" w305 {
          tunnel: w304 -> [_ w309]
          tunnel: w303 -> [_ w306]
          frame False {
          }
          frame True {
            n195 = vi-ref "校准任务设置.vi"() -> (w312:refnum<vi>)
            n196 = property class="VI"(reference=w312) -> (reference out=w308:refnum<vi>, "Name"=w310:string, "Exec.State"=w311:T10)  [unwired: 1 in, 1 out]
            n197 = case shown="\"Idle\"" w311 {
              tunnel: w310 -> [_ w322]
              tunnel: w309 -> [_ w317]
              tunnel: w308 -> [w313 w314]
              tunnel: [w313 w314] -> w307
              frame "Bad", Default {
              }
              frame "Idle" {
                n198 = Open VI Reference(type specifier VI Refnum (for type only)=refnum<vi> refnum ("类型说明符VI引用句柄（仅用于类型）"), vi path=w322, options=128 ("选项")) -> (vi reference=w319:refnum<vi>, error out=w318:errorcluster)  [unwired: 3 in]
                n199 = call-by-ref "开始异步调用"(reference=w319, error in=w318, "用户事件"=w317) -> (reference out=w316:refnum<vi>, error out=w315:errorcluster)  [unwired: 11 in]
                n200 = Close Reference(reference=w316, error in (no error)=w315) -> ()  [unwired: 1 out]
              }
            }
            n201 = invoke on="子面板" class="SubPnl" method="Insert VI"(error in=w306, "VI Ref"=w307) -> ()  [unwired: 2 in, 4 out]
          }
        }
      }
      event "校准按钮": Value Change {
        n202 = event-data() -> ("CtlRef"=w325:refnum<vi>, "NewVal"=w327:T1)  [unwired: 1 in, 4 out]
        n203 = Not Equal?(x=w327, y=T1."未选择") -> (x != y?=w328:bool)
        n204 = case shown="真" w328 {
          tunnel: w331 -> [_ w339]
          tunnel: w330 -> [_ w337]
          tunnel: w327 -> [_ w341]
          tunnel: w326 -> [_ _]
          tunnel: w325 -> [_ _]
          tunnel: w324 -> [_ _]
          tunnel: w323 -> [_ w340]
          frame False {
          }
          frame True {
            (unwired) u16 21 items=["CODMn"=21] ("参数下拉列表")
            n205 = property class="Enum (严格)"(reference=w337) -> ("Value"=w336:enum16{"低量程", "高量程"})  [unwired: 1 in, 2 out]
            n206 = property class="Ring (严格)"(reference=w339) -> ("Value"=w338:u16)  [unwired: 1 in, 2 out]
            n207 = local read "曲线模型"() -> (w334:T3)
            n208 = case shown="\"跨度核查\"" w341 {
              tunnel: w334 -> [_ w343 w345 w346 w348 w350]
              tunnel: [_ w342 w344 w347 w349 w351] -> w333
              frame "未选择", Default {
              }
              frame "空白校准" {
                n209 = Unbundle By Name(w343) -> ("标液浓度1"=w342:dbl)
              }
              frame "标样校准" {
                n210 = Unbundle By Name(w345) -> ("标液浓度2"=w344:dbl)
              }
              frame "标样核查" {
                n211 = Unbundle By Name(w346) -> ("标液浓度3"=w347:dbl)
              }
              frame "零点核查" {
                n212 = Unbundle By Name(w348) -> ("标液浓度4"=w349:dbl)
              }
              frame "跨度核查" {
                n213 = Unbundle By Name(w350) -> ("标液浓度5"=w351:dbl)
              }
            }
            n214 = Bundle By Name(cluster=T5 {"id"=0, "任务类型"=enum."未选择", "量程下拉列表"=enum."低量程", "状态"=enum."待执行", "标液浓度"=0.0, "吸光值"=0.0, "校准时间"=timestamp(0 s since 1904-01-01), "报警状态"=enum."正常数据"} ("校准任务"), "id"=w338, "任务类型"=w341, "量程下拉列表"=w336, "标液浓度"=w333) -> (w335:T5)
            n215 = Generate User Event(user event=w340, event data cluster=w335) -> ()  [unwired: 2 in, 2 out]
          }
        }
      }
      event "历史数据导入": Value Change {
        n216 = event-data() -> ("NewVal"=w354:T1)  [unwired: 1 in, 5 out]
        n217 = Not Equal?(x=w354, y=T1."未选择") -> (x != y?=w355:bool)
        n218 = case shown="真" w355 {
          tunnel: w358 -> [_ w368]
          tunnel: w357 -> [_ w367]
          tunnel: w354 -> [_ w361]
          tunnel: w353 -> [_ _]
          tunnel: w352 -> [_ w365]
          frame False {
          }
          frame True {
            n219 = property class="Enum (严格)"(reference=w367) -> ("Value"=w363:enum16{"低量程", "高量程"})  [unwired: 1 in, 2 out]
            n220 = property class="Ring (严格)"(reference=w368) -> ("Value"=w364:u16)  [unwired: 1 in, 2 out]
            n221 = property on="历史数据导入" class="RadioBtnsControl (严格)"("Value"=T1."未选择" ("历史数据导入")) -> ()  [unwired: 2 in, 2 out]
            n222 = call "校准数据选择表.vi"("历史数据导入"=w361, "量程下拉列表"=w363, "table"="CODMn") -> ("布尔"=w366:bool, "输出"=w359:T11)  [unwired: 7 in]
            n223 = case shown="真" w366 {
              tunnel: w359 -> [_ w374]
              tunnel: w365 -> [_ w378]
              tunnel: w364 -> [_ w375]
              tunnel: w363 -> [_ w373]
              tunnel: w361 -> [_ w372]
              frame False {
              }
              frame True {
                n224 = Unbundle By Name(w374) -> ("标液值"=w371:dbl, "吸光值"=w370:dbl, "时间"=w369:timestamp)
                n225 = Bundle By Name(cluster=T5 {"id"=0, "任务类型"=enum."未选择", "量程下拉列表"=enum."低量程", "状态"=enum."已执行", "标液浓度"=0.0, "吸光值"=0.0, "校准时间"=timestamp(0 s since 1904-01-01), "报警状态"=enum."正常数据"} ("事件数据"), "id"=w375, "任务类型"=w372, "量程下拉列表"=w373, "标液浓度"=w371, "吸光值"=w370, "校准时间"=w369) -> (w376:T5)
                n226 = Generate User Event(user event=w378, event data cluster=w376) -> ()  [unwired: 2 in, 2 out]
              }
            }
          }
        }
      }
    }
  }
